vi "Set to State.vi"(8 "error in":errorcluster, 10 "State":T1, 11 "Data in":T2={"Class"={"Ants"=refnum, "Layer"=refnum, "Templates"=refnum, "Icon"=refnum, "Glyph"=refnum, "Settings"=refnum, "Tools"=refnum, "History"=refnum}, "Ref"={"Add Layer"=refnum, "Remove Layer"=refnum, "Line Text"=[], "Body Text Spec"=refnum, "DNL_Font"=refnum, "glyph path str"=refnum, "templates path str"=refnum, "Arrow Up"=refnum, "Arrow Down"=refnum, "IE VI Ref"=refnum, "Glyphs tree"=refnum, "Templates tree"=refnum, "Layer Icon Text"=refnum, "Layer Template"=refnum, "Body Text"=refnum, "Search Templates"=refnum, "TextMarker"=refnum, "Tab Control"=refnum, "Search Glyphs"=refnum, "Line Color"=refnum, "DNL_Glyphs []"=refnum, "Fill Color"=refnum, "Tools"=refnum, "Icon"=refnum, "Preview"=refnum, "Ants"=refnum, "Terminals"=refnum, "menu reference"=refnum, "LayerNames"=[], "GlyphLoadAnimation"=refnum, "TemplateLoadAnimation"=refnum, "refreshGlyphs"=refnum, "refreshTemplates"=refnum}, "Support"={"AntsRect"={"left"=0, "top"=0, "right"=0, "bottom"=0}, "Mouse Move Coords"={"Horizontal"=0, "Vertical"=0}, "Mouse Down Coords"={"Horizontal"=0, "Vertical"=0}, "Temp Coord"={"Horizontal"=0, "Vertical"=0}, "Action"=enum."Default", "Edge Color"=4914962, "Fill Color"=16860, "Mouse Down?"=FALSE, "Draft Mode?"=FALSE, "Temp Icon"=bytes[3102], "CTRL Pressed"=FALSE, "Move Selection?"=FALSE, "AntsRect Orig"={"left"=0, "top"=0, "right"=0, "bottom"=0}, "Text"="", "TM Set?"=FALSE, "Mouse inside icon?"=FALSE, "Tool (old value)"=0, "Pencil Move Color"=0, "Swap Colors?"=FALSE, "Shift pressed?"=FALSE}}) -> (0 "error out":errorcluster, 3 "Data out":T2={"Class"={"Ants"=refnum, "Layer"=refnum, "Templates"=refnum, "Icon"=refnum, "Glyph"=refnum, "Settings"=refnum, "Tools"=refnum, "History"=refnum}, "Ref"={"Add Layer"=refnum, "Remove Layer"=refnum, "Line Text"=[], "Body Text Spec"=refnum, "DNL_Font"=refnum, "glyph path str"=refnum, "templates path str"=refnum, "Arrow Up"=refnum, "Arrow Down"=refnum, "IE VI Ref"=refnum, "Glyphs tree"=refnum, "Templates tree"=refnum, "Layer Icon Text"=refnum, "Layer Template"=refnum, "Body Text"=refnum, "Search Templates"=refnum, "TextMarker"=refnum, "Tab Control"=refnum, "Search Glyphs"=refnum, "Line Color"=refnum, "DNL_Glyphs []"=refnum, "Fill Color"=refnum, "Tools"=refnum, "Icon"=refnum, "Preview"=refnum, "Ants"=refnum, "Terminals"=refnum, "menu reference"=refnum, "LayerNames"=[], "GlyphLoadAnimation"=refnum, "TemplateLoadAnimation"=refnum, "refreshGlyphs"=refnum, "refreshTemplates"=refnum}, "Support"={"AntsRect"={"left"=0, "top"=0, "right"=0, "bottom"=0}, "Mouse Move Coords"={"Horizontal"=0, "Vertical"=0}, "Mouse Down Coords"={"Horizontal"=0, "Vertical"=0}, "Temp Coord"={"Horizontal"=0, "Vertical"=0}, "Action"=enum."Default", "Edge Color"=4914962, "Fill Color"=16860, "Mouse Down?"=FALSE, "Draft Mode?"=FALSE, "Temp Icon"=bytes[3102], "CTRL Pressed"=FALSE, "Move Selection?"=FALSE, "AntsRect Orig"={"left"=0, "top"=0, "right"=0, "bottom"=0}, "Text"="", "TM Set?"=FALSE, "Mouse inside icon?"=FALSE, "Tool (old value)"=0, "Pencil Move Color"=0, "Swap Colors?"=FALSE, "Shift pressed?"=FALSE}})   [LabVIEW 2020, in "lv_icon.lvlib" / "History.lvlib"]
uses:
  History.lvlib
  Class/Ants/Ants.lvclass
  Class/FakedArray/FakedArray.lvclass
  vi.lib/LabVIEW Icon API/lv_icon/Classes/Icon/Icon.lvclass
  Class/Icon Library/Glyph.lvclass
  Class/Settings/Settings.lvclass
  Class/Tools/Tools Paint.lvclass
  History/History.lvclass
  vi.lib/LabVIEW Icon API/lv_icon/Controls/Layer.ctl
  649d0eb5-19f0-431c-9115-02f03f72a685.vi
  vi.lib/LabVIEW Icon API/lv_icon/Controls/Font.ctl
  vi.lib/LabVIEW Icon API/lv_icon/Controls/Alignment.ctl
  vi.lib/LabVIEW Icon API/lv_icon/Controls/BodyText.ctl
  vi.lib/LabVIEW Icon API/lv_icon/Controls/Graphic.ctl
  <vilib>/Utility/miscctls.llb/LVPoint32TypeDef.ctl
  Controls/SupportClass_Action.ctl
  vi.lib/LabVIEW Icon API/lv_icon/Controls/IEColor.ctl
  Controls/Support Cluster.ctl
  lv_icon.lvlib
  Controls/References Cluster.ctl
  Controls/IE Classes.ctl
  Controls/Global Data.ctl
  State.ctl
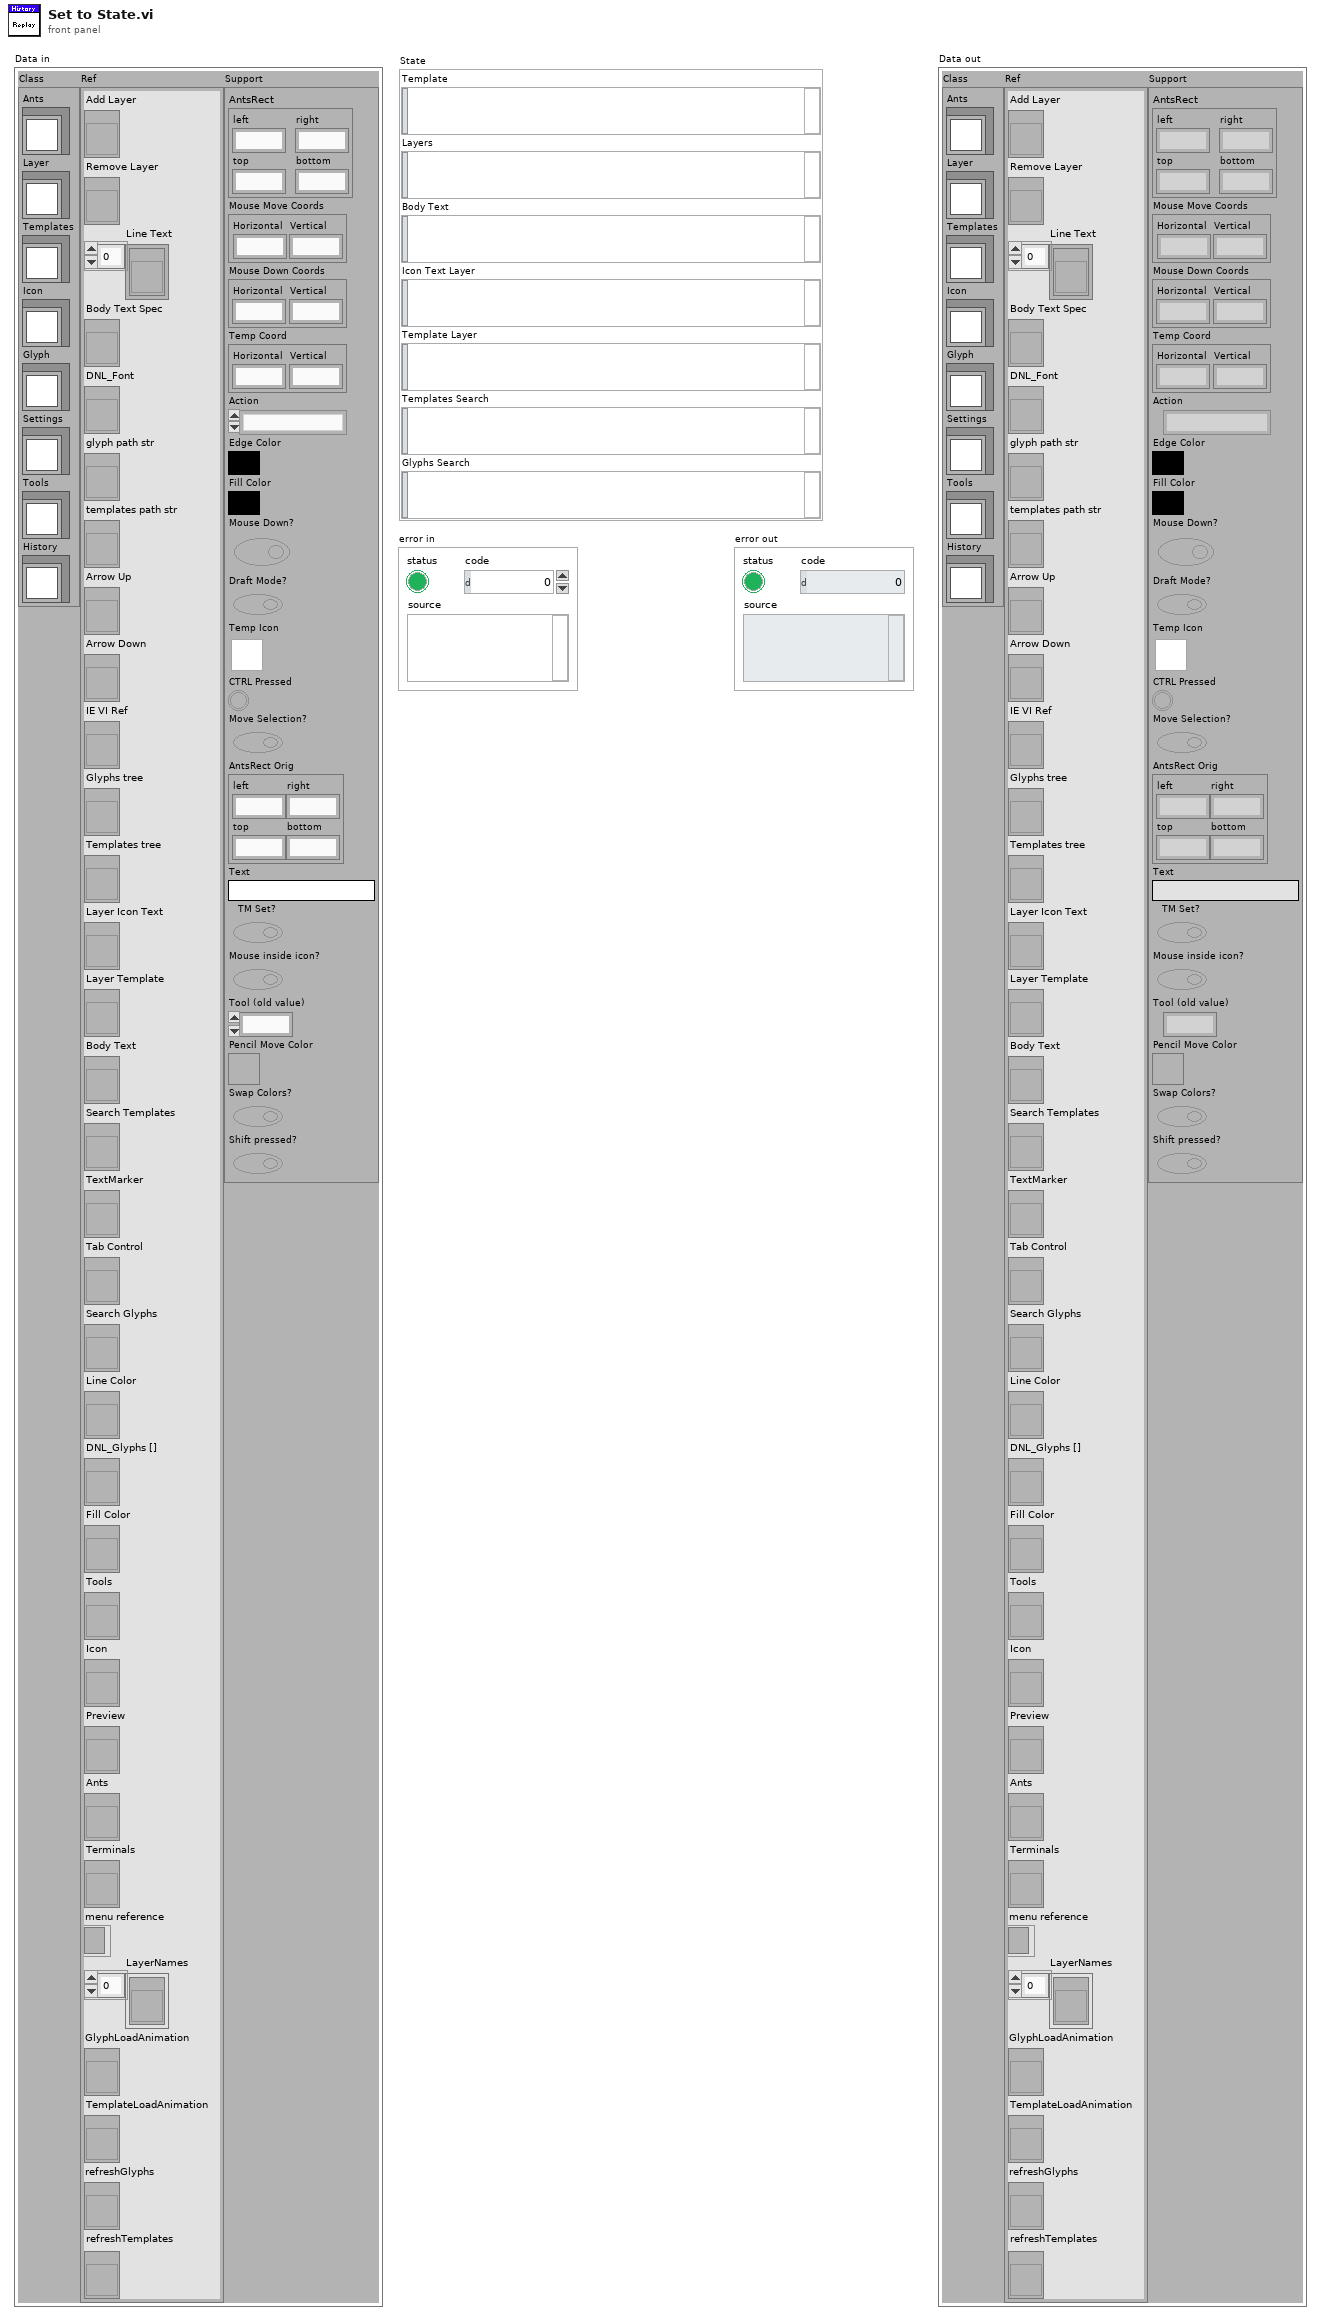
[diagram p1: front panel]
types:
  T1 = typedef "lv_icon.lvlib/History.lvlib/State.ctl" = cluster{"Template":string, "Layers":string, "Body Text":string, "Icon Text Layer":string, "Template Layer":string, "Templates Search":string, "Glyphs Search":string}
  T2 = typedef "lv_icon.lvlib/Global Data.ctl" = cluster{"Class":T3, "Ref":T4, "Support":T5}
  T3 = typedef "lv_icon.lvlib/IE Classes.ctl" = cluster{"Ants":refnum<class "Ants.lvclass">, "Layer":refnum<class "FakedArray.lvclass">, "Templates":refnum<class "FakedArray.lvclass">, "Icon":refnum<class "Icon.lvclass">, "Glyph":refnum<class "Glyph.lvclass">, "Settings":refnum<class "Settings.lvclass">, "Tools":refnum<class "Tools Paint.lvclass">, "History":refnum<class "History.lvclass">}
  T4 = typedef "lv_icon.lvlib/References Cluster.ctl" = cluster{"Add Layer":refnum<vi>, "Remove Layer":refnum<vi>, "Line Text":refnum<vi>[], "Body Text Spec":refnum<vi>, "DNL_Font":refnum<vi>, "glyph path str":refnum<vi>, "templates path str":refnum<vi>, "Arrow Up":refnum<vi>, "Arrow Down":refnum<vi>, "IE VI Ref":refnum<vi>, "Glyphs tree":refnum<vi>, "Templates tree":refnum<vi>, "Layer Icon Text":refnum<vi>, "Layer Template":refnum<vi>, "Body Text":refnum<vi>, "Search Templates":refnum<vi>, "TextMarker":refnum<vi>, "Tab Control":refnum<vi>, "Search Glyphs":refnum<vi>, "Line Color":refnum<vi>, "DNL_Glyphs []":refnum<vi>, "Fill Color":refnum<vi>, "Tools":refnum<vi>, "Icon":refnum<vi>, "Preview":refnum<vi>, "Ants":refnum<vi>, "Terminals":refnum<vi>, "menu reference":refnum<k9>, "LayerNames":refnum<vi>[], "GlyphLoadAnimation":refnum<vi>, "TemplateLoadAnimation":refnum<vi>, "refreshGlyphs":refnum<vi>, "refreshTemplates":refnum<vi>}
  T5 = typedef "lv_icon.lvlib/Support Cluster.ctl" = cluster{"AntsRect":cluster{"left":i16, "top":i16, "right":i16, "bottom":i16}, "Mouse Move Coords":T6, "Mouse Down Coords":T6, "Temp Coord":T6, "Action":T7, "Edge Color":T8, "Fill Color":T8, "Mouse Down?":bool, "Draft Mode?":bool, "Temp Icon":picture, "CTRL Pressed":bool, "Move Selection?":bool, "AntsRect Orig":cluster{"left":i16, "top":i16, "right":i16, "bottom":i16}, "Text":string, "TM Set?":bool, "Mouse inside icon?":bool, "Tool (old value)":u32, "Pencil Move Color":u32, "Swap Colors?":bool, "Shift pressed?":bool}
  T6 = typedef "LVPoint32TypeDef.ctl" = cluster{"Horizontal":i32, "Vertical":i32}
  T7 = typedef "SupportClass_Action.ctl" = enum16{"Default", "Move Selection", "Glyph Library", "Tool"}
  T8 = typedef "IEColor.ctl" = u32
  T9 = enum8{"Glyphs Search", "Templates Search", "Templates Tree", "Template Layer", "Icon Text Layer", "Body Text", "Layers", "Template"}
  T10 = enum8{"Glyphs Search", "Templates Search", "Templates Tree", "Template Layer", "Icon Text Layer", "Body Text", "Layers", "Template"}[]
  T11 = typedef "Layer.ctl" = cluster{"LayerIcon":picture, "LayerName":string, "Opacity":u8, "Visibility?":bool}
  T12 = typedef "BodyText.ctl" = cluster{"Line 1 text":string, "Line 2 text":string, "Line 3 text":string, "Line 4 text":string, "Line 1 color":u32, "Line 2 color":u32, "Line 3 color":u32, "Line 4 color":u32, "Body Text Spec":cluster{"Font":T13, "Alignment":T14, "Size":u8}, "Center text vertically":bool, "Capitalize Text":bool}
  T13 = typedef "Font.ctl" = string
  T14 = typedef "Alignment.ctl" = u16
  T15 = typedef "Graphic.ctl" = cluster{"Rectangle":cluster{"left":i16, "top":i16, "right":i16, "bottom":i16}, "Path":path, "Image":picture, "Filter":string, "FileName":string}
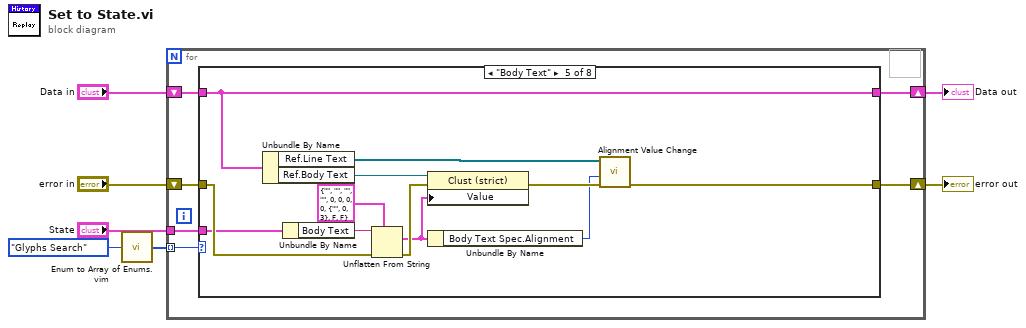
[diagram p0: block diagram]
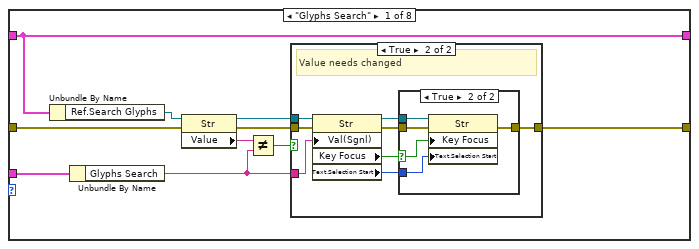
[diagram p2: hidden frame]
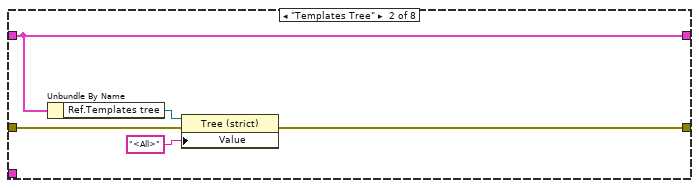
[diagram p5: hidden frame]
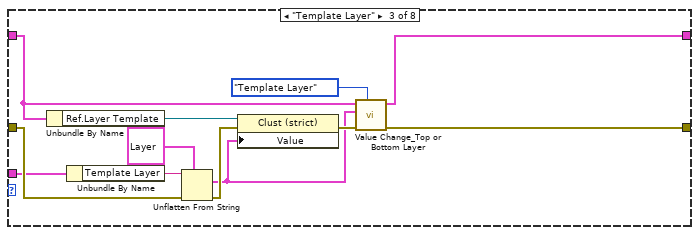
[diagram p6: hidden frame]
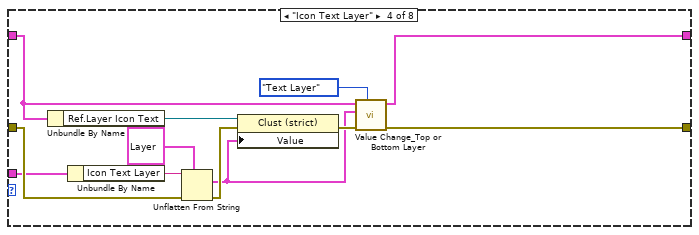
[diagram p7: hidden frame]
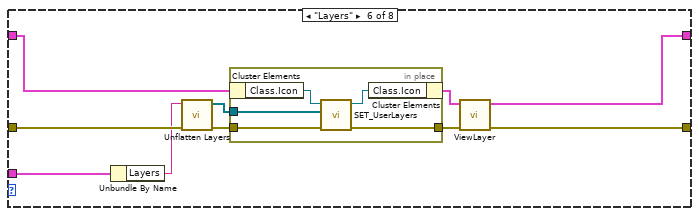
[diagram p8: hidden frame]
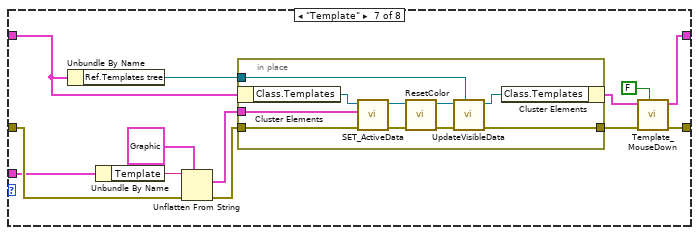
[diagram p9: hidden frame]
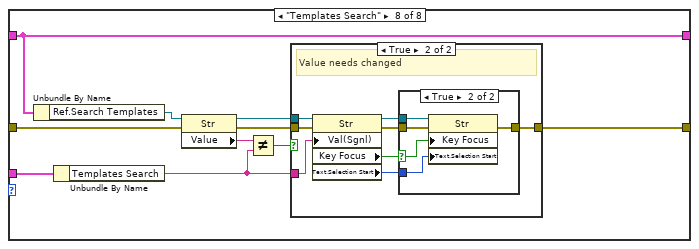
[diagram p10: hidden frame]
diagram:
  n1 = call "Enum to Array of Enums.vim"("enum"=T9."Glyphs Search") -> ("array of enums"=w4:T10)
  n2 = for "Natt Sequence - http://bit.ly/nattsequence" {
    tunnel: w4 -> [w11] mode=indexing
    shift-right: [w12] -> w6
    shift-left: "error in" -> [w13]
    shift-right: [w9] -> w1
    shift-left: "Data in" -> [w10]
    tunnel: "State" -> [w8]
    n3 = case shown="\"Body Text\"" w11 {
      tunnel: w13 -> [w23 w43 w53 w65 w79 w87 w105 w127]
      tunnel: w10 -> [w20 w40 w44 w56 w77 w81 w96 w124]
      tunnel: [w20 w40 w45 w57 w77 w82 w97 w124] -> w9
      tunnel: w8 -> [w19 _ w47 w59 w76 w85 w99 w123]
      tunnel: [w21 w42 w52 w64 w70 w86 w104 w125] -> w12
      frame "Glyphs Search" {
        n4 = Unbundle By Name(w20) -> ("Ref.Search Glyphs"=w18:refnum<vi>)
        n5 = Unbundle By Name(w19) -> ("Glyphs Search"=w15:string)
        n6 = property class="Str"(reference=w18, error in=w23) -> (reference out=w17:refnum<vi>, error out=w22:errorcluster, "Value"=w16:string)
        n7 = Not Equal?(x=w16, y=w15) -> (x != y?=w14:bool)
        n8 = case shown="True" w14 {
          tunnel: w15 -> [_ w29]
          tunnel: w17 -> [_ w28]
          tunnel: w22 -> [w24 w32]
          tunnel: [w24 w30] -> w21
          frame False {
            # "Value does not need changed"
          }
          frame True {
            # "Value needs changed"
            n9 = property class="Str"(reference=w28, error in=w32, "Val(Sgnl)"=w29) -> (reference out=w25:refnum<vi>, error out=w31:errorcluster, "Key Focus"=w27:bool, "Text.Selection Start"=w26:u32)
            n10 = case shown="True" w27 {
              selector: w27 -> [_ w35]
              tunnel: w26 -> [_ w36]
              tunnel: w25 -> [_ w34]
              tunnel: w31 -> [w33 w38]
              tunnel: [w33 w37] -> w30
              frame False {
              }
              frame True {
                n11 = property class="Str"(reference=w34, error in=w38, "Key Focus"=w35, "Text.Selection Start"=w36) -> (error out=w37:errorcluster)  [unwired: 1 out]
              }
            }
          }
        }
      }
      frame "Templates Tree" {
        n12 = Unbundle By Name(w40) -> ("Ref.Templates tree"=w39:refnum<vi>)
        n13 = property class="Tree (strict)"(reference=w39, error in=w43, "Value"="<All>") -> (error out=w42:errorcluster)  [unwired: 1 out]
      }
      frame "Template Layer" {
        n14 = Unbundle By Name(w44) -> ("Ref.Layer Template"=w48:refnum<vi>)
        n15 = Unbundle By Name(w47) -> ("Template Layer"=w46:string)
        n16 = Unflatten From String(type=T11 {"LayerIcon"=bytes[3102], "LayerName"="", "Opacity"=100, "Visibility?"=TRUE}, binary string=w46, error in (no error)=w53) -> (value=w51:T11, error out=w55:errorcluster)  [unwired: 3 out]
        n17 = property class="Clust (strict)"(reference=w48, error in=w55, "Value"=w51) -> (error out=w54:errorcluster)  [unwired: 1 out]
        n18 = call "Value Change_Top or Bottom Layer.vi"("Type"=enum16{"Template Layer", "Text Layer"}."Template Layer", "error in (no error)"=w54, "Data"=w51, "Data in"=w44) -> ("error out"=w52:errorcluster, "Data out"=w45:T2)  [unwired: 6 out]
      }
      frame "Icon Text Layer" {
        n19 = Unbundle By Name(w56) -> ("Ref.Layer Icon Text"=w60:refnum<vi>)
        n20 = Unbundle By Name(w59) -> ("Icon Text Layer"=w58:string)
        n21 = Unflatten From String(type=T11 {"LayerIcon"=bytes[3102], "LayerName"="", "Opacity"=100, "Visibility?"=TRUE}, binary string=w58, error in (no error)=w65) -> (value=w63:T11, error out=w67:errorcluster)  [unwired: 3 out]
        n22 = property class="Clust (strict)"(reference=w60, error in=w67, "Value"=w63) -> (error out=w66:errorcluster)  [unwired: 1 out]
        n23 = call "Value Change_Top or Bottom Layer.vi"("Type"=enum16{"Template Layer", "Text Layer"}."Text Layer", "error in (no error)"=w66, "Data"=w63, "Data in"=w56) -> ("error out"=w64:errorcluster, "Data out"=w57:T2)  [unwired: 6 out]
      }
      frame "Body Text" {
        n24 = Unbundle By Name(w77) -> ("Ref.Line Text"=w72:refnum<vi>[], "Ref.Body Text"=w73:refnum<vi>)
        n25 = Unbundle By Name(w76) -> ("Body Text"=w75:string)
        n26 = Unflatten From String(type=T12 {"Line 1 text"="", "Line 2 text"="", "Line 3 text"="", "Line 4 text"="", "Line 1 color"=0, "Line 2 color"=0, "Line 3 color"=0, "Line 4 color"=0, "Body Text Spec"={"Font"="", "Alignment"=0, "Size"=3}, "Center text vertically"=FALSE, "Capitalize Text"=FALSE} ("Body Text 2"), binary string=w75, error in (no error)=w79) -> (value=w69:T12, error out=w78:errorcluster)  [unwired: 1 in, 2 out]
        n27 = property class="Clust (strict)"(reference=w73, error in=w78, "Value"=w69) -> (error out=w71:errorcluster)  [unwired: 1 out]
        n28 = Unbundle By Name(w69) -> ("Body Text Spec.Alignment"=w68:T14)
        n29 = call "Alignment Value Change.vi"("error in"=w71, "NewVal"=w68, "Line Text"=w72) -> ("error out"=w70:errorcluster)  [unwired: 2 in, 6 out]
      }
      frame "Layers" {
        n30 = Unbundle By Name(w85) -> ("Layers"=w83:string)
        n31 = call "Unflatten Layers.vi"("Error In"=w87, "String"=w83) -> ("Error Out"=w89:errorcluster, "Layers"=w84:refnum<class "Layer.lvclass">[])  [unwired: 8 in]
        n32 = in-place {
          in-place-border: w84 -> [w92]
          in-place-border: w89 -> [w94]
          in-place-border: [w93] -> w88
          n33 = in-place-cluster #1(w81) -> ("Class.Icon"=w91:refnum<class "Icon.lvclass">)
          n34 = call-dynamic "SET_UserLayers.vi"("error in (no error)"=w94, "Layers"=w92, "Icon.lvclass in"=w91) -> ("error out"=w93:errorcluster, "Icon.lvclass out"=w90:refnum<class "Icon.lvclass">)  [unwired: 7 in]
          n35 = in-place-cluster #1("Class.Icon"=w90) -> (w80:T2)
        }
        n36 = call "ViewLayer.vi"("error in (no error)"=w88, "Data in"=w80) -> ("error out"=w86:errorcluster, "Data out"=w82:T2)  [unwired: 2 in, 6 out]
      }
      frame "Template" {
        n37 = Unbundle By Name(w96) -> ("Ref.Templates tree"=w103:refnum<vi>)
        n38 = Unbundle By Name(w99) -> ("Template"=w98:string)
        n39 = Unflatten From String(type=T15 {"Rectangle"={"left"=0, "top"=0, "right"=0, "bottom"=0}, "Path"=path "", "Image"=bytes[0], "Filter"="", "FileName"=""}, binary string=w98, error in (no error)=w105) -> (value=w101:T15, error out=w106:errorcluster)  [unwired: 3 out]
        n40 = in-place {
          in-place-border: w103 -> [w113]
          in-place-border: [w117] -> w107
          in-place-border: w106 -> [w116]
          in-place-border: w101 -> [w110]
          n41 = in-place-cluster #2(w96) -> ("Class.Templates"=w109:refnum<class "FakedArray.lvclass">)
          n42 = call-dynamic "SET_ActiveData.vi"("error in (no error)"=w116, "Active Data"=w110, "FakedArray.lvclass in"=w109) -> ("error out"=w115:errorcluster, "FakedArray.lvclass out"=w112:refnum<class "FakedArray.lvclass">)  [unwired: 7 out]
          n43 = call "ResetColor.vi"("error in (no error)"=w115, "FakedArray in"=w112) -> ("error out"=w114:errorcluster, "FakedArray out"=w111:refnum<class "FakedArray.lvclass">)  [unwired: 8 out]
          n44 = call-dynamic "UpdateVisibleData.vi"("Templates tree"=w113, "error in (no error)"=w114, "FakedArray in"=w111) -> ("error out"=w117:errorcluster, "FakedArray out"=w108:refnum<class "FakedArray.lvclass">)  [unwired: 2 in, 5 out]
          n45 = in-place-cluster #2("Class.Templates"=w108) -> (w95:T2)
        }
        n46 = call "Template_MouseDown.vi"("Add to Undo?"=FALSE, "error in"=w107, "Data in"=w95) -> ("error out"=w104:errorcluster, "Data out"=w97:T2)  [unwired: 2 in, 5 out]
      }
      frame "Templates Search" {
        n47 = Unbundle By Name(w124) -> ("Ref.Search Templates"=w122:refnum<vi>)
        n48 = Unbundle By Name(w123) -> ("Templates Search"=w119:string)
        n49 = property class="Str"(reference=w122, error in=w127) -> (reference out=w121:refnum<vi>, error out=w126:errorcluster, "Value"=w120:string)
        n50 = Not Equal?(x=w120, y=w119) -> (x != y?=w118:bool)
        n51 = case shown="True" w118 {
          tunnel: w119 -> [_ w133]
          tunnel: w121 -> [_ w132]
          tunnel: w126 -> [w128 w136]
          tunnel: [w128 w134] -> w125
          frame False {
            # "Value does not need changed"
          }
          frame True {
            # "Value needs changed"
            n52 = property class="Str"(reference=w132, error in=w136, "Val(Sgnl)"=w133) -> (reference out=w129:refnum<vi>, error out=w135:errorcluster, "Key Focus"=w131:bool, "Text.Selection Start"=w130:u32)
            n53 = case shown="True" w131 {
              selector: w131 -> [_ w139]
              tunnel: w130 -> [_ w140]
              tunnel: w129 -> [_ w138]
              tunnel: w135 -> [w137 w142]
              tunnel: [w137 w141] -> w134
              frame False {
              }
              frame True {
                n54 = property class="Str"(reference=w138, error in=w142, "Key Focus"=w139, "Text.Selection Start"=w140) -> (error out=w141:errorcluster)  [unwired: 1 out]
              }
            }
          }
        }
      }
    }
  }
  "Data out" <- w1
  "error out" <- w6
